vi "GetLastChar.vi"(10 "String":string) -> (2 "String 2":string)   [LabVIEW 2013]
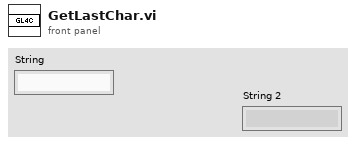
[diagram p1: front panel]
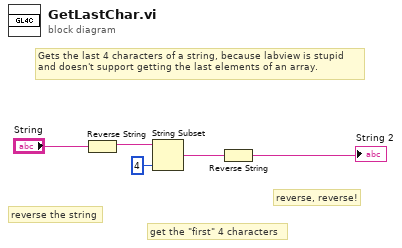
[diagram p0: block diagram]
diagram:
  # "reverse, reverse!"
  # "get the \"first\" 4 characters"
  # "reverse the string"
  # "Gets the last 4 characters of a string, because labview is stupid\nand doesn't support getting the last elements of an array."
  n1 = Reverse String(1:"String") -> (0:w3:string)
  n2 = String Subset(string=w3, length (rest)=4 ("length (rest)")) -> (substring=w2:string)  [unwired: 1 in]
  n3 = Reverse String(1:w2) -> (0:→"String 2":string)
